vi "Extract Port From Host String.vi"(0 "host in":string) -> (4 "host out":string, 6 "port":u16, 8 "found?":bool)   [LabVIEW 2014, in "AMC.lvlib"]
uses:
  AMC.lvlib
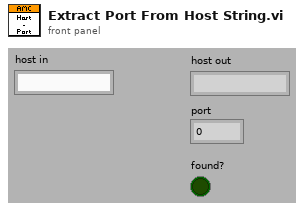
[diagram p1: front panel]
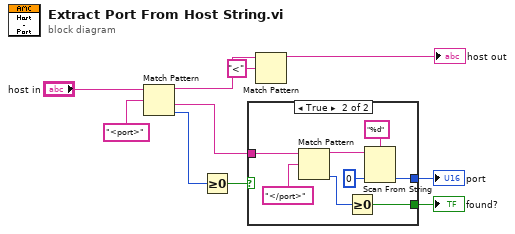
[diagram p0: block diagram]
diagram:
  n1 = Match Pattern(string="host in", regular expression="<port>" ("string")) -> (before substring=w3:string, after substring=w10:string, offset past match=w9:i32)  [unwired: 1 in, 1 out]
  n2 = Greater Or Equal To 0?(x=w9) -> (x >= 0?=w8:bool)
  n3 = case shown="True" w8 {
    tunnel: w10 -> [_ w14]
    tunnel: [_ w13] -> w5
    tunnel: [_ w11] -> w4
    frame False {
    }
    frame True {
      n4 = Match Pattern(string=w14, regular expression="</port>" ("string")) -> (before substring=w16:string, offset past match=w12:i32)  [unwired: 1 in, 2 out]
      n5 = Greater Or Equal To 0?(x=w12) -> (x >= 0?=w11:bool)
      n6 = Scan From String(format string="%d", input string=w16, default 1=u16 0 ("default value 1")) -> (output 1=w13:u16)  [unwired: 2 in, 3 out]
    }
  }
  "port" <- w5
  "found?" <- w4
  n7 = Match Pattern(string=w3, regular expression="<") -> (before substring=→"host out":string)  [unwired: 1 in, 3 out]
